vi "Select_a_Channel.vi"(6 "Mode":T1(ring), 7 "Extra channel names":string[](array[string]), 8 "Data Filename":path) -> (0 "Current Values":string[](array[string]), 1 "Channel Values":string[](array[string]), 2 "Selected Channel Names":string[](array[string]), 3 "Data Filename Out":path)   [LabVIEW 2010]
uses:
  ADAM Client/Sub VIs/ADAM Controls/Channel_names.ctl
  ADAM Client/Sub VIs/ADAM Controls/Calib_type_ADAM.ctl
panel:
  in  "Tolerance":dbl=1.0 format="%.4f"
  in  "OK":bool
  in  "Search String":string
  in  "Listbox":i32[](listbox)
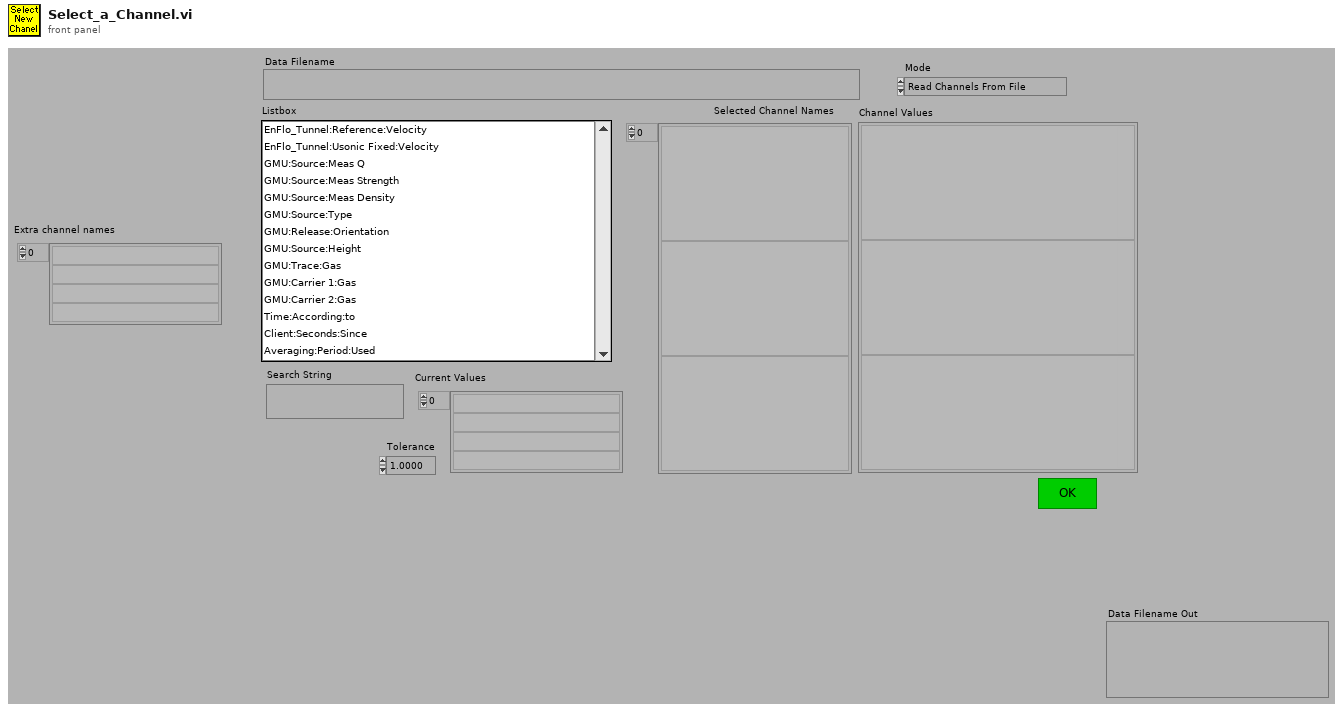
[diagram p1: front panel]
types:
  T1 = enum16{"Read Channels From File", "Read Channels from Server"}
  T2 = typedef "Channel_names.ctl" = enum16{"Active Only", "Active + Off", "All Channels"}
  T3 = typedef "Calib_type_ADAM.ctl" = enum16{"Raw", "Bx + A", "Cx^2 + Bx + A", "Dx^3 + Cx^2 + Bx + A", "In Band", "Hi-Tec Q", "Hi-Tec M_dot", "Text"}
  T4 = enum32{"existing file", "new file", "new or existing file", "existing dir", "new dir", "new or existing dir", "existing file (use LLBs)", "new file (use LLBs)", "new or existing file (use LLBs)", "new or existing file or directory (use LLBs)"}
  T5 = typedef "Ch_description_ADAM.ctl" = cluster{"Ch Name":string, "Type":T6, "Function":T7, "Ch State":T8, "Calibration type":T3, "A":dbl, "B":dbl, "C":dbl, "D":dbl, "Comments":string, "Address":T9, "String":string, "Duty":u16}
  T6 = typedef "Module_type_ADAM.ctl" = enum16{"4011", "4012", "4013", "4014", "4016", "4017", "4018", "4021", "4050", "4052", "4053", "4060", "4080", "5000", "5017", "5018", "5024", "5051", "5056", "5060", "6060", "Tracker", "WEST", "GILL", "JEM", "VICI", "Vaisala", "DRUCK", "Run VI Named:", "IR2100", "PPT", "Comparator", "VIRTUAL", "Hold Value", "Read A", "Read Ch", "Coded", "Client Info", "Web Client", "X10", "Test"}
  T7 = typedef "Function_ADAM.ctl" = enum16{"Analogue Input", "Digital Input", "Event counter", "Event rate", "Analogue Output", "Digital Output", "Relay Output"}
  T8 = typedef "Channel_State.ctl" = enum16{"On", "Off", "Always On", "Always Off"}
  T9 = typedef "Address.ctl" = cluster{"Main":i32, "Ch.":i32, "Sub":i32, "Port Name":string}
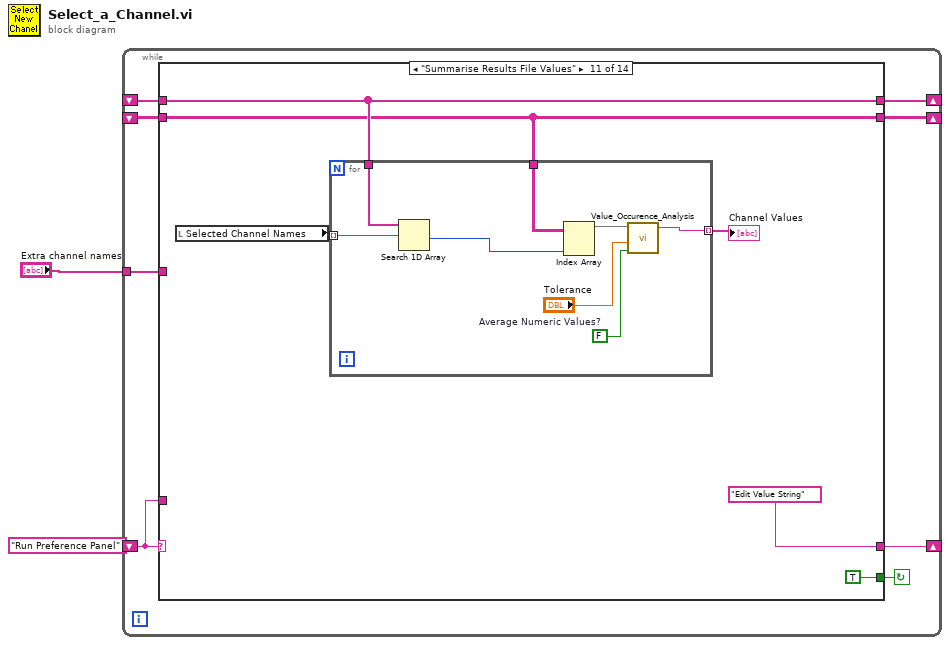
[diagram p0: block diagram]
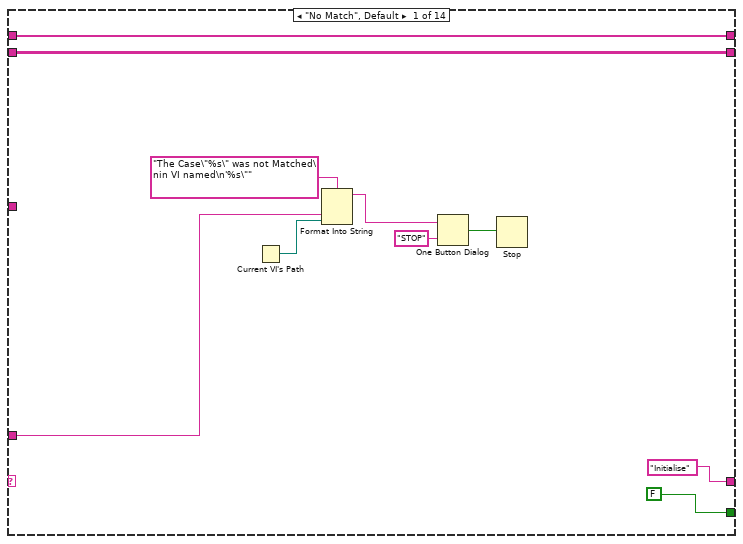
[diagram p2: hidden frame]
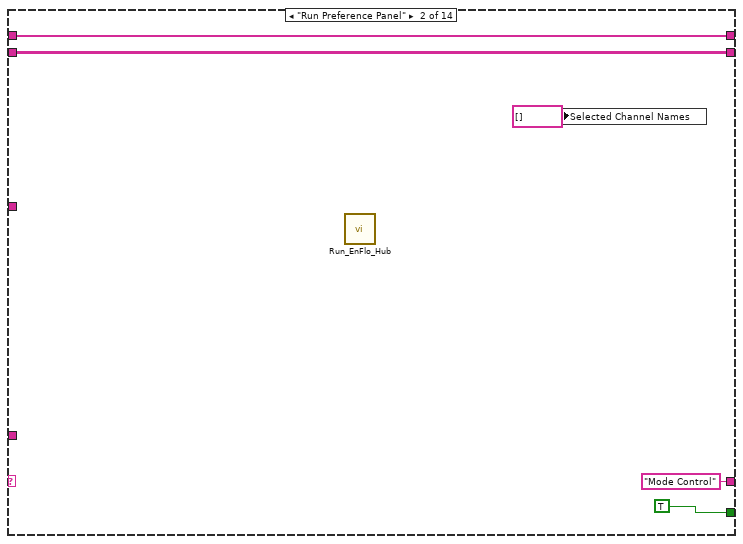
[diagram p3: hidden frame]
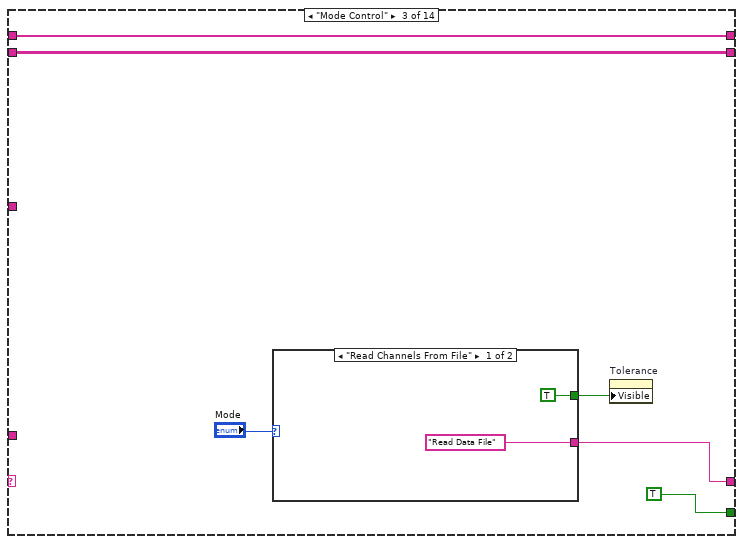
[diagram p4: hidden frame]
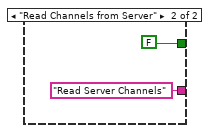
[diagram p5: hidden frame]
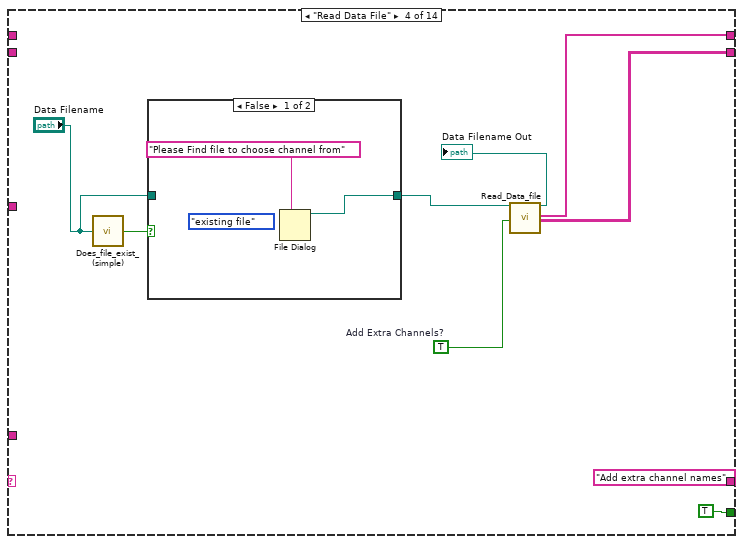
[diagram p6: hidden frame]
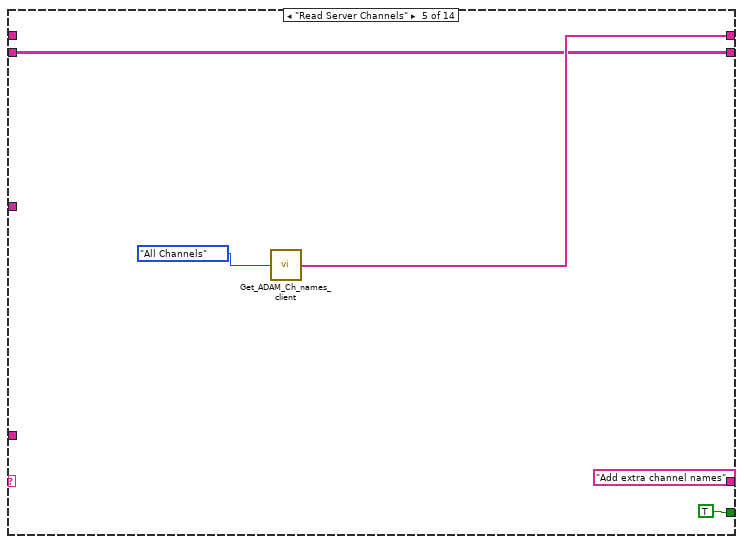
[diagram p8: hidden frame]
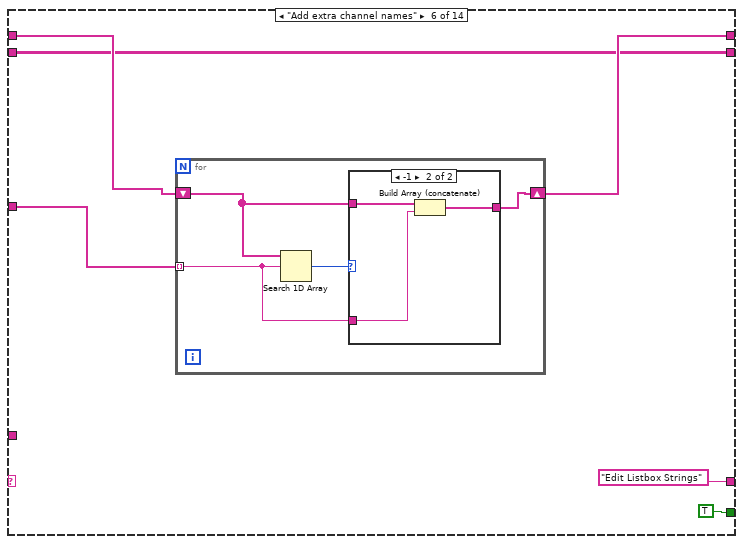
[diagram p9: hidden frame]
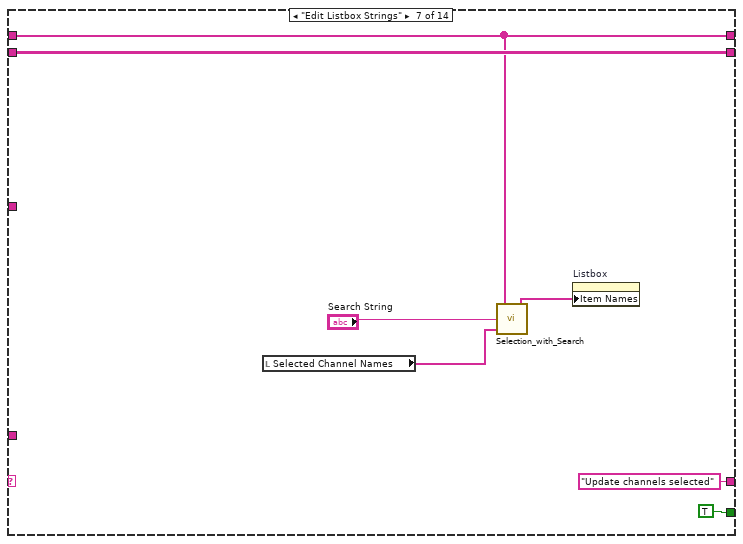
[diagram p11: hidden frame]
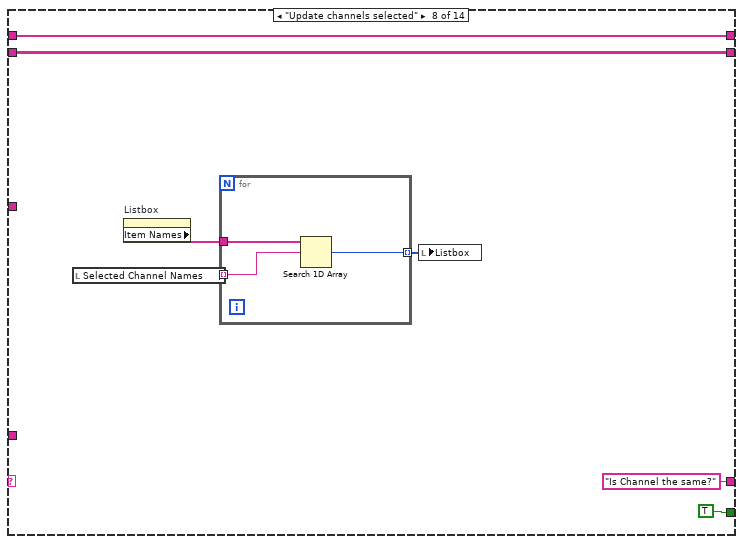
[diagram p12: hidden frame]
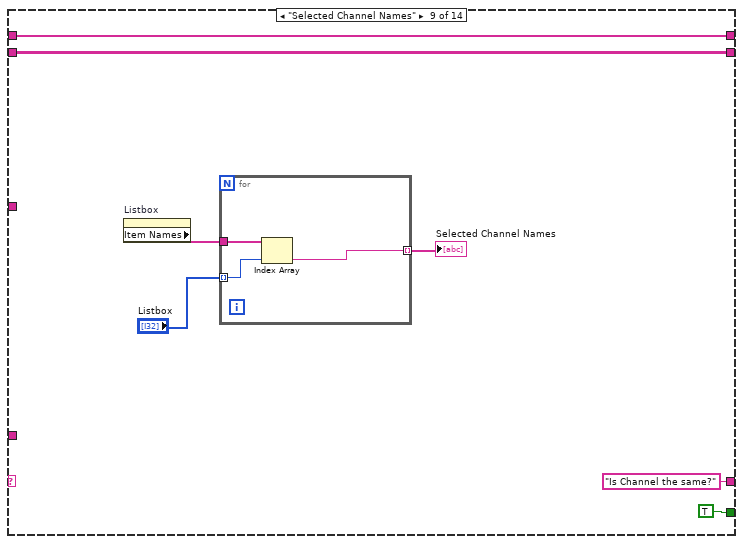
[diagram p13: hidden frame]
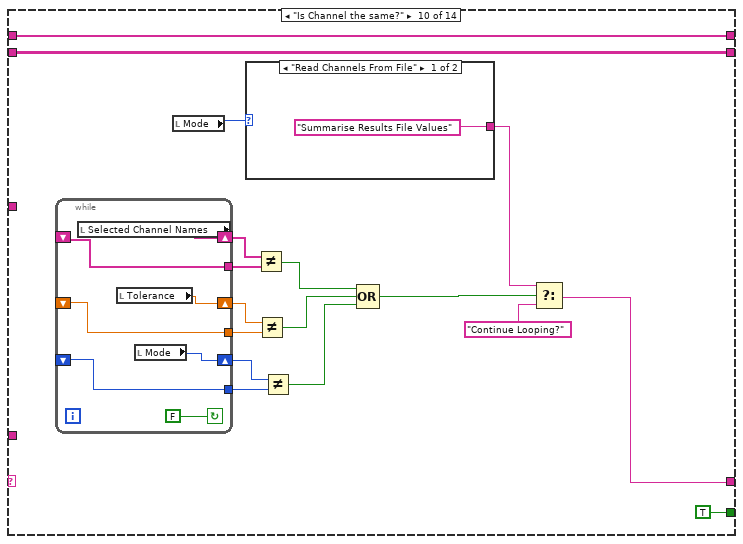
[diagram p14: hidden frame]
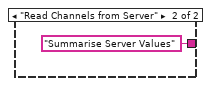
[diagram p15: hidden frame]
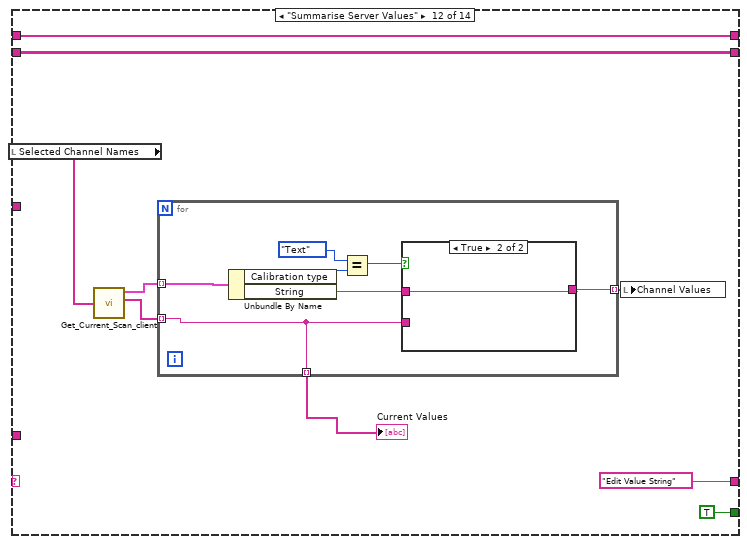
[diagram p16: hidden frame]
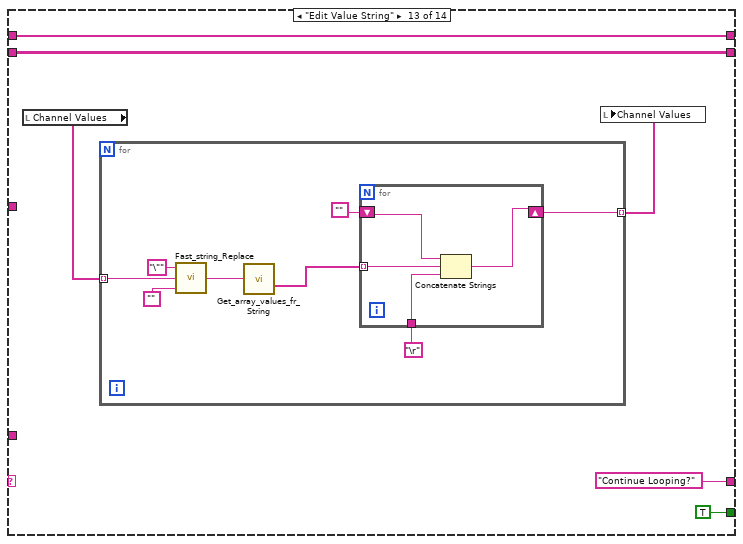
[diagram p18: hidden frame]
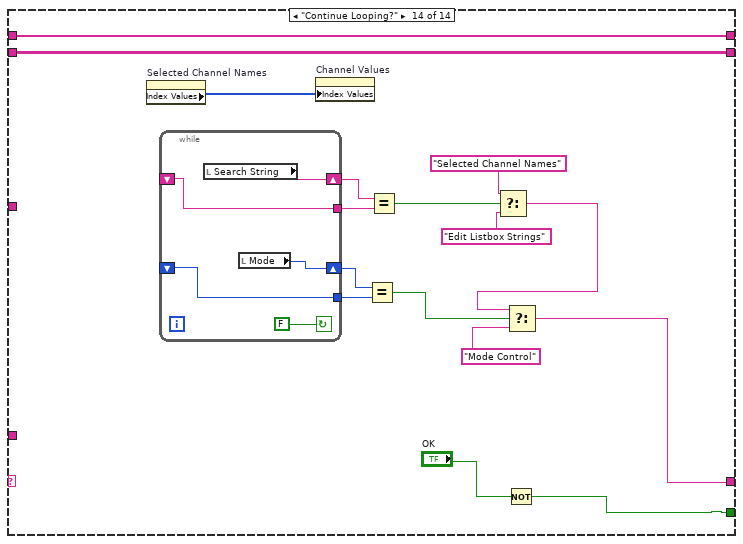
[diagram p19: hidden frame]
diagram:
  n1 = while {
    shift-left: _ -> [w4]
    shift-right: [w6] -> _
    shift-left: _ -> [w5]
    shift-right: [w7] -> _
    shift-left: "Run Preference Panel" -> [w8]
    shift-right: [w9] -> _
    tunnel: "Extra channel names" -> [w3]
    stop <- w10 continue-if-true
    n2 = case shown="\"Summarise Results File Values\"" w8 {
      tunnel: [FALSE TRUE TRUE TRUE TRUE TRUE TRUE TRUE TRUE TRUE TRUE TRUE TRUE w182] -> w10
      tunnel: ["Initialise" "Mode Control" w28 "Add extra channel names" "Add extra channel names" "Edit Listbox Strings" "Update channels selected" "Is Channel the same?" "Is Channel the same?" w105 "Edit Value String" "Edit Value String" "Continue Looping?" w177] -> w9
      tunnel: w8 -> [w15 _ _ _ _ _ _ _ _ _ _ _ _ _]
      tunnel: [w12 w24 w30 w42 w50 w54 w71 w78 w88 w108 w124 w139 w154 w185] -> w7
      tunnel: [w11 w23 w29 w41 w49 w53 w72 w79 w89 w109 w122 w140 w155 w184] -> w6
      tunnel: w5 -> [w12 w24 w30 _ _ w56 w71 w78 w88 w108 w124 w139 w154 w185]
      tunnel: w4 -> [w11 w23 w29 _ w49 w53 w72 w79 w89 w109 w122 w140 w155 w184]
      tunnel: w3 -> [_ _ _ _ _ w55 _ _ _ _ _ _ _ _]
      frame "No Match", Default {
        n3 = Current VI's Path() -> (path=w14:path)
        n4 = Format Into String(format string="The Case\"%s\" was not Matched\nin VI named\n'%s\"" ("Format String"), w15, w14) -> (resulting string=w18:string)  [unwired: 2 in, 1 out]
        n5 = One Button Dialog(message=w18, button name ("OK")="STOP") -> (true=w16:bool)
        n6 = Stop(stop? (T)=w16) -> ()
      }
      frame "Run Preference Panel" {
        n7 = call "Run_EnFlo_Hub.vi"() -> ()  [unwired: 8 out]
        n8 = local write "Selected Channel Names"(string[] [] ("Selected Channel Names")) -> ()
      }
      frame "Mode Control" {
        n9 = case shown="\"Read Channels From File\"" "Mode" {
          tunnel: ["Read Data File" "Read Server Channels"] -> w28
          tunnel: [TRUE FALSE] -> w27
          frame "Read Channels From File" {
          }
          frame "Read Channels from Server" {
          }
        }
        n10 = property on="Tolerance" class="DigNum (strict)"("Visible"=w27) -> ()  [unwired: 2 in, 2 out]
      }
      frame "Read Data File" {
        w40 = TRUE  # Add Extra Channels?
        n11 = call "Does_file_exist_(simple).vi"("Pathname"="Data Filename") -> ("exists?"=w39:bool)
        n12 = case shown="False" w39 {
          tunnel: [w46 w47] -> w37
          tunnel: "Data Filename" -> [_ w47]
          frame False {
            (unwired) T4."existing file" ("select mode (2)")
            n13 = File Dialog(7:"Please Find file to choose channel from" ("prompt")) -> (3:w46:path)  [unwired: 1 in, 8 out]
          }
          frame True {
          }
        }
        n14 = call "Read_Data_file.vi"("Results file"=w37, "Add Extra Channels?"=w40) -> ("Results file Out"=→"Data Filename Out":path, "Ch names Out"=w42:string[], "Channel Values Out"=w41:string[][])  [unwired: 3 in, 12 out]
      }
      frame "Read Server Channels" {
        n15 = call "Get_ADAM_Ch_names_client.vi"("Channel names set"=Channel_names."All Channels") -> ("Ch names"=w50:string[])
      }
      frame "Add extra channel names" {
        n16 = for {
          shift-right: [w60] -> w54
          shift-left: w56 -> [w61]
          tunnel: w55 -> [w59] mode=indexing
          n17 = Search 1D Array(1D array=w61, element=w59) -> (index of element=w62:i32)  [unwired: 1 out]
          n18 = case shown="-1" w62 {
            tunnel: w61 -> [w63 w66]
            tunnel: [w63 w65] -> w60
            tunnel: w59 -> [_ w64]
            frame 0, Default {
            }
            frame -1 {
              n19 = Build Array (concatenate)(w66, w64) -> (w65:string[])
            }
          }
        }
      }
      frame "Edit Listbox Strings" {
        n20 = local read "Selected Channel Names"() -> (w67:string[])
        n21 = call "Selection_with_Search.vi"("Selected Channel Names"=w67, "Search String"="Search String", "All Channel Names"=w71) -> ("Item Names"=w68:string[])
        n22 = property on="Listbox" class="LstBox (strict)"("Item Names"=w68) -> ()  [unwired: 2 in, 2 out]
      }
      frame "Update channels selected" {
        n23 = local read "Selected Channel Names"() -> (w75:string[])
        n24 = property on="Listbox" class="LstBox (strict)"() -> ("Item Names"=w76:string[])  [unwired: 2 in, 2 out]
        n25 = for {
          tunnel: w76 -> [w83]
          tunnel: w75 -> [w82] mode=indexing
          tunnel: [w81] -> w74 mode=indexing
          n26 = Search 1D Array(1D array=w83, element=w82) -> (index of element=w81:i32)  [unwired: 1 out]
        }
        n27 = local write "Listbox"(w74) -> ()
      }
      frame "Selected Channel Names" {
        n28 = property on="Listbox" class="LstBox (strict)"() -> ("Item Names"=w86:string[])  [unwired: 2 in, 2 out]
        n29 = for {
          tunnel: w86 -> [w93]
          tunnel: "Listbox" -> [w92] mode=indexing
          tunnel: [w91] -> w84 mode=indexing
          n30 = Index Array(array=w93, index=w92) -> (element=w91:string)
        }
        "Selected Channel Names" <- w84
      }
      frame "Is Channel the same?" {
        n31 = while {
          tunnel: [w113] -> w97
          shift-left: _ -> [w113]
          shift-right: [w112] -> w98
          tunnel: [w114] -> w104
          shift-left: _ -> [w114]
          shift-right: [w115] -> w103
          tunnel: [w116] -> w106
          shift-left: _ -> [w116]
          shift-right: [w117] -> w107
          stop <- FALSE continue-if-true
          n32 = local read "Selected Channel Names"() -> (w117:string[])
          n33 = local read "Tolerance"() -> (w115:dbl)
          n34 = local read "Mode"() -> (w112:T1)
        }
        n35 = local read "Mode"() -> (w99:T1)
        n36 = case shown="\"Read Channels From File\"" w99 {
          tunnel: ["Summarise Results File Values" "Summarise Server Values"] -> w95
          frame "Read Channels From File" {
          }
          frame "Read Channels from Server" {
          }
        }
        n37 = Not Equal?(x=w107, y=w106) -> (x != y?=w102:bool)
        n38 = Not Equal?(x=w103, y=w104) -> (x != y?=w101:bool)
        n39 = Not Equal?(x=w98, y=w97) -> (x != y?=w96:bool)
        n40 = Compound Arithmetic op=OR(w102, w101, w96) -> (w100:bool)
        n41 = Select(t=w95, s=w100, f="Continue Looping?") -> (s? t:f=w105:string)
      }
      frame "Summarise Results File Values" {
        n42 = local read "Selected Channel Names"() -> (w123:string[])
        n43 = for {
          tunnel: w124 -> [w133]
          tunnel: w123 -> [w132] mode=indexing
          tunnel: w122 -> [w130]
          tunnel: [w127] -> w120 mode=indexing
          w126 = FALSE  # Average Numeric Values?
          n44 = Search 1D Array(1D array=w133, element=w132) -> (index of element=w131:i32)  [unwired: 1 out]
          n45 = Index Array(array=w130, index (col)=w131) -> (element=w129:string[])  [unwired: 1 in]
          n46 = call "Value_Occurence_Analysis.vi"("Average Numeric Values?"=w126, "Tolerance"="Tolerance", "String Array"=w129) -> ("Output String"=w127:string)  [unwired: 1 in, 2 out]
        }
        "Channel Values" <- w120
      }
      frame "Summarise Server Values" {
        n47 = local read "Selected Channel Names"() -> (w138:string[])
        n48 = call "Get_Current_Scan_client.vi"("ADAM Ch Names"=w138) -> ("Ch Description Array"=w137:T5[], "String values"=w136:string[])  [unwired: 2 out]
        n49 = for {
          tunnel: w137 -> [w144] mode=indexing
          tunnel: w136 -> [w143] mode=indexing
          tunnel: [w145] -> w134 mode=indexing
          tunnel: [w143] -> w135 mode=indexing
          n50 = Unbundle By Name(w144) -> ("Calibration type"=w149:T3, "String"=w146:string)
          n51 = Equal?(x=Calib_type_ADAM."Text" ("Calibration Type"), y=w149) -> (x = y?=w147:bool)
          n52 = case shown="True" w147 {
            tunnel: [w150 w151] -> w145
            tunnel: w146 -> [_ w151]
            tunnel: w143 -> [w150 _]
            frame False {
            }
            frame True {
            }
          }
        }
        "Current Values" <- w135
        n53 = local write "Channel Values"(w134) -> ()
      }
      frame "Edit Value String" {
        n54 = local read "Channel Values"() -> (w153:string[])
        n55 = for {
          tunnel: w153 -> [w159] mode=indexing
          tunnel: [w158] -> w152 mode=indexing
          n56 = call "Fast_string_Replace.vi"("Replace match with:"="", "Input String"=w159, "regular expression"="\"") -> ("Output String"=w160:string)  [unwired: 2 out]
          n57 = call "Get_array_values_fr_String.vi"("String Value"=w160) -> ("String array"=w165:string[])  [unwired: 1 out]
          n58 = for {
            shift-right: [w166] -> w158
            shift-left: "" -> [w169]
            tunnel: w165 -> [w168] mode=indexing
            tunnel: "\r" -> [w167]
            n59 = Concatenate Strings(w169, w168, w167) -> (w166:string)
          }
        }
        n60 = local write "Channel Values"(w152) -> ()
      }
      frame "Continue Looping?" {
        n61 = property on="Selected Channel Names" class="Arr (strict)"() -> ("Index Values"=w170:u32[])  [unwired: 2 in, 2 out]
        n62 = while {
          tunnel: [w187] -> w176
          shift-left: _ -> [w187]
          shift-right: [w188] -> w175
          tunnel: [w190] -> w180
          shift-left: _ -> [w190]
          shift-right: [w189] -> w181
          stop <- FALSE continue-if-true
          n63 = local read "Search String"() -> (w188:string)
          n64 = local read "Mode"() -> (w189:T1)
        }
        n65 = property on="Channel Values" class="Arr (strict)"("Index Values"=w170) -> ()  [unwired: 2 in, 2 out]
        n66 = Equal?(x=w181, y=w180) -> (x = y?=w179:bool)
        n67 = Equal?(x=w175, y=w176) -> (x = y?=w174:bool)
        n68 = Select(t="Selected Channel Names", s=w174, f="Edit Listbox Strings") -> (s? t:f=w171:string)
        n69 = Not(x="OK") -> (.not. x?=w182:bool)
        n70 = Select(t=w171, s=w179, f="Mode Control") -> (s? t:f=w177:string)
      }
    }
  }
